vi "Dummy.vi"(8 "error in (no error)":errorcluster, 11 "Dummy in":refnum<class "Dummy.lvclass">) -> (0 "error out":errorcluster, 3 "Dummy out":refnum<class "Dummy.lvclass">)   [LabVIEW 2009, in "Dummy.lvclass"]
uses:
  Dummy.lvclass
  Readable/Channel Names.ctl
  Readable/Readable.lvclass
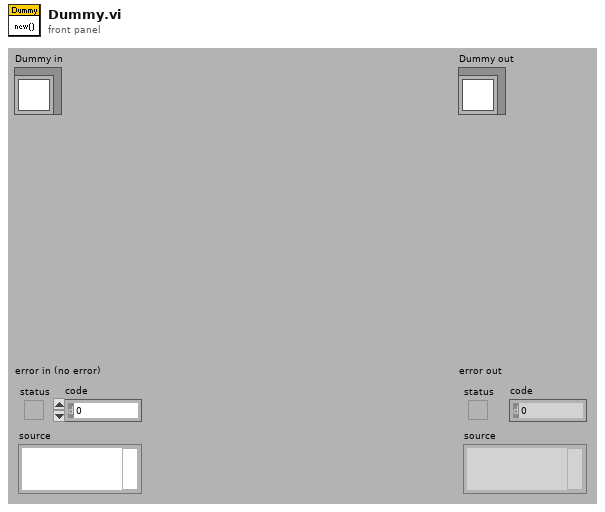
[diagram p1: front panel]
types:
  T1 = typedef "Readable.lvclass/Channel Names.ctl" = string[]
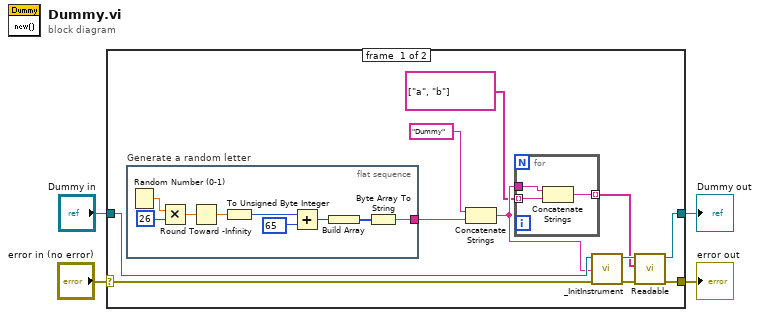
[diagram p0: block diagram]
diagram:
  n1 = case shown="No Error" "error in (no error)" {
    selector: "error in (no error)" -> [w14 w29]
    tunnel: [w9 w29] -> w3
    tunnel: [w8 w28] -> w1
    tunnel: "Dummy in" -> [w15 w28]
    frame #0 {
      n2 = flat-sequence "Generate a random letter" {
        tunnel: [w19] -> w13
        frame #0 {
          n3 = Random Number (0-1)() -> (number: 0 to 1=w26:dbl)
          n4 = Multiply(x=w26, y=u8 26) -> (x*y=w25:dbl)
          n5 = Round Toward -Infinity(1:w25) -> (0:w21:dbl)
          n6 = To Unsigned Byte Integer(number=w21) -> (unsigned 8bit integer=w20:u8)
          n7 = Add(x=w20, y=u8 65) -> (x+y=w23:u8)
          n8 = Build Array(w23) -> (w22:u8[])
          n9 = Byte Array To String(unsigned byte array=w22) -> (string=w19:string)
        }
      }
      n10 = Concatenate Strings("Dummy", w13) -> (w7:string)
      n11 = for {
        tunnel: w7 -> [w18]
        tunnel: T1 ["a", "b"] ("Channel Names") -> [w17] mode=indexing
        tunnel: [w16] -> w5 mode=indexing
        n12 = Concatenate Strings(w18, w17) -> (w16:string)
      }
      n13 = call-dynamic "_InitInstrument.vi"("error in (no error)"=w14, "Name"=w7, "Instrument in"=w15) -> ("error out"=w10:errorcluster, "Instrument out"=w11:refnum<class "Dummy.lvclass">)  [unwired: 3 in, 4 out]
      n14 = call "Readable.vi"("error in (no error)"=w10, "Channel Names"=w5, "Readable in"=w11) -> ("error out"=w9:errorcluster, "Readable out"=w8:refnum<class "Dummy.lvclass">)  [unwired: 7 in]
    }
    frame #1 {
    }
  }
  "error out" <- w3
  "Dummy out" <- w1
